vi "Get Tip From WRL.vi"(8 "error in (no error)":errorcluster, 11 "Tip Model File (.wrl)":path) -> (0 "error out":errorcluster, 3 "SceneObject out":refnum<vi>)   [LabVIEW 2013]
doc: "This VI loads a tip from a WRL (3D model file) and scales it appropriately."
uses:
  <vilib>/picture/3D Picture Control/NI_3D Picture Control.lvlib
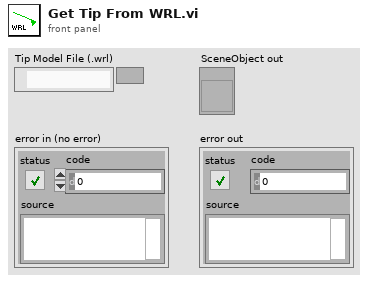
[diagram p1: front panel]
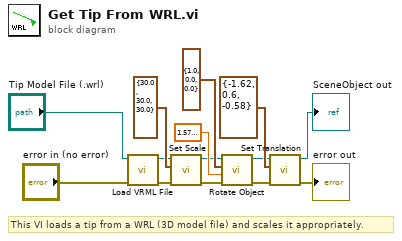
[diagram p0: block diagram]
diagram:
  # "This VI loads a tip from a WRL (3D model file) and scales it appropriately."
  n1 = call <vilib>:"Load VRML File.vi"("error in"="error in (no error)", "Path"="Tip Model File (.wrl)") -> ("error out"=w7:errorcluster, "Scene:Read Scene File"=w6:refnum<vi>)  [unwired: 8 in]
  n2 = call <vilib>:"Set Scale.vi"("error in (no error)"=w7, "Scale"=cluster{"X":dbl, "Y":dbl, "Z":dbl} {"X"=30.0, "Y"=30.0, "Z"=30.0} ("Scaling Factor"), "Scene Object"=w6) -> ("error out"=w8:errorcluster, "Scaled Object"=w3:refnum<vi>)  [unwired: 7 in]
  n3 = call <vilib>:"Rotate Object.vi"("error in (no error)"=w8, "Angle"=sgl 1.57, "Axis"=cluster{"X":sgl, "Y":sgl, "Z":sgl} {"X"=1.0, "Y"=0.0, "Z"=0.0}, "Scene.Object In"=w3) -> ("error out"=w9:errorcluster, "Scene.Object Out"=w2:refnum<vi>)  [unwired: 6 in]
  n4 = call <vilib>:"Set Translation.vi"("error in (no error)"=w9, "Translation"=cluster{"X":dbl, "Y":dbl, "Z":dbl} {"X"=-1.62, "Y"=0.6, "Z"=-0.58} ("Initial Coordinate"), "Scene Object"=w2) -> ("error out"=→"error out":errorcluster, "Translated Object"=→"SceneObject out":refnum<vi>)  [unwired: 7 in]
